vi "DPT Call.vi"() -> ()   [LabVIEW 2014]
panel:
  in  "Source Library Path":path=path "\\\\192.168.1.12\\share/AP1_Library/Executables/Dryer Performance Test"
  out "Array 2":bool[](array[boolean])=[TRUE, TRUE, TRUE, TRUE]
  out "Error Array":errorcluster[](array[cluster])
  out "Response":string[](array[string])
  out "Cmd":i32
  in  "error in (no error)":errorcluster
  out "Cmds Array":string[](array[string])
  in  "configuration file path":path=path "C:/work/DryerPerformanceTest.ini"
  in  "data backup command line":string="robocopy \"c:\\Data\" \"XXX\"  /XN"
  in  "update command line":string="robocopy \"XXX\"  \"c:\\Program Files\\GE\\Dryer Performance Test\" /XN"
  in  "backup command line":string="robocopy \"c:\\Program Files\\GE\\Dryer Performance Test\"  \"c:\\Program Files\\GE\\backup\" /XN"
  out "error out":errorcluster
  in  "command line":string="\"c:\\Program Files\\GE\\Dryer Performance Test\\Dryer Performance Test.exe\""
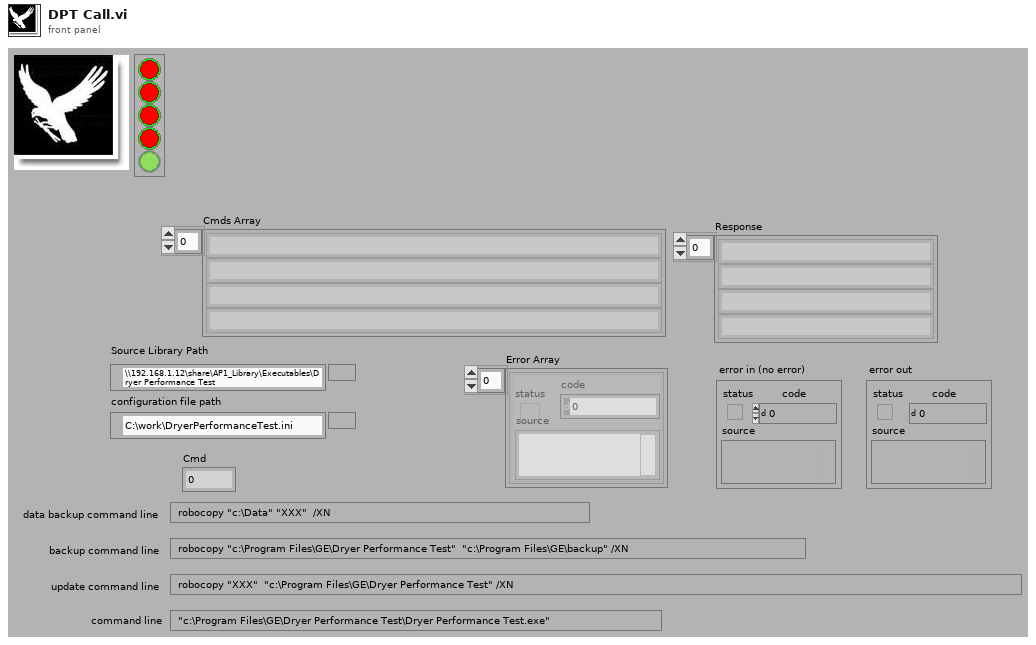
[diagram p1: front panel]
types:
  T1 = typedef "DPT Global Type.ctl" = cluster{"Test Setup":cluster{"RH Resistor":dbl, "Temp Cal":dbl, "Temp Coeff":dbl, "Power On Threshold":dbl, "MA Filter Size":i32, "Weight Offset":dbl, "Temp Resistor":dbl, "Gas Enabled":bool, "Gas P. Resistor":dbl, "Scale Com":dbl, "W. Samps":i32, "Temp4mA Val":dbl, "Temp20mA Val":dbl, "RH4mA Val":dbl, "RH20mA Val":dbl, "GPres4mA Val":dbl, "Gpres20mA Val":dbl, "Smoothing":bool, "CDAQ":bool, "34970":bool, "34980":bool, "RH-IP":string, "RH-IP2":string, "RH-IP3":string, "CompVolume":dbl, "T45_Coeff.":dbl}, "Agilent Setup":cluster{"Scale Channel":string, "TC Channels":string, "VDC Discrete Channels":string, "RH Chan":string, "Temp Chan":string, "Tscale Channel":string, "RDB Channel":string, "Gas Temperature":string, "Gas Pressure":string, "Barometric Pressure":string, "Gas Feedback Chan":string}, "Directories":cluster{"Work File Directory":path, "Save File Directory":path, "Library Directory":path, "Data Backup Directory":path, "Data Backup Dir Fail":path, "Lab Directory":path}, "Test Information":cluster{"Model:":string, "Temperature:":string, "Engineer:":string, "Technician:":string, "Comments:":string, "Lab ID:":string, "TR Number:":string, "Test Number:":string, "Test Station:":string, "Empty Dryer Cold Weight:":dbl, "Serial Number:":string, "Build:":string, "Dryer Type":string, "Humidity":string, "Test Title per TR:":string}, "cDAQ Array Locations":cluster{"Scale Channel":string, "TC Channels":string, "VDC Discrete Channel":string, "RH Chan":string, "Temp Chan":string, "Tscale Channel":string, "RDB Channel":string, "Gas Temperature":string, "Gas Pressure":string, "Barometric Pressure":string, "Gas Feedback Chan":string}}
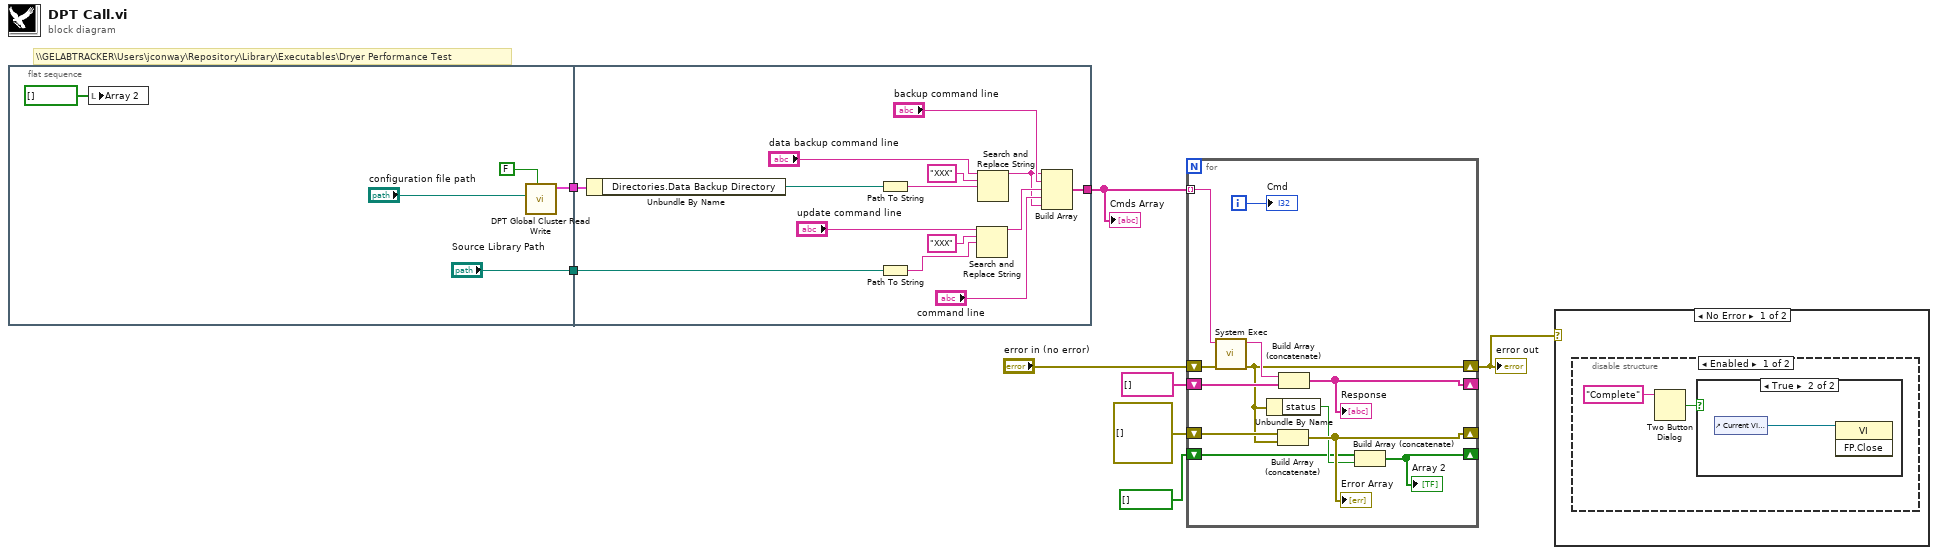
[diagram p0: block diagram]
diagram:
  # "\\\\GELABTRACKER\\Users\\jconway\\Repository\\Library\\Executables\\Dryer Performance Test"
  n1 = flat-sequence {
    tunnel: [w13] -> w7
    tunnel: ["Source Library Path"] -> w1
    tunnel: [w26] -> w8
    tunnel: w7 -> [w23]
    tunnel: w1 -> [w14]
    frame #0 {
      n2 = local write "Array 2"(bool[] [] ("Array 2")) -> ()
      n3 = call "DPT Global Cluster Read Write.vi"("Write?"=FALSE, "configuration file path"="configuration file path") -> ("Test Config Out"=w13:T1)  [unwired: 8 in, 1 out]
    }
    frame #1 {
      n4 = Unbundle By Name(w23) -> ("Directories.Data Backup Directory"=w25:path)
      n5 = Path To String(path=w25) -> (string=w24:string)
      n6 = Path To String(path=w14) -> (string=w20:string)
      n7 = Search and Replace String(input string="update command line", search string="XXX", replace string=w20) -> (result string=w16:string)  [unwired: 5 in, 3 out]
      n8 = Search and Replace String(input string="data backup command line", search string="XXX", replace string=w24) -> (result string=w15:string)  [unwired: 5 in, 3 out]
      n9 = Build Array(w15, "backup command line", w16, "command line", w15) -> (w26:string[])
    }
  }
  n10 = for {
    tunnel: w8 -> [w39] mode=indexing
    shift-right: [w32] -> w5
    shift-left: "error in (no error)" -> [w38]
    shift-right: [w34] -> _
    shift-left: string[] [] -> [w35]
    shift-right: [w31] -> _
    shift-left: errorcluster[] [] -> [w33]
    shift-right: [w28] -> _
    shift-left: bool[] [] -> [w29]
    i -> [w37]
    n11 = call <vilib>:"System Exec.vi"("error in (no error)"=w38, "command line"=w39) -> ("error out"=w32:errorcluster, "standard output"=w36:string)  [unwired: 6 in, 2 out]
    n12 = Unbundle By Name(w32) -> ("status"=w30:bool)
    n13 = Build Array (concatenate)(w33, w32) -> (w31:errorcluster[])
    "Error Array" <- w31
    n14 = Build Array (concatenate)(w36, w35) -> (w34:string[])
    "Response" <- w34
    n15 = Build Array (concatenate)(w29, w30) -> (w28:bool[])
    "Array 2" <- w28
    "Cmd" <- w37
  }
  "error out" <- w5
  n16 = case shown="No Error" w5 {
    frame No Error {
      n17 = disable-structure shown="Enabled" {
        frame Enabled {
          n18 = Two Button Dialog(message="Complete") -> (T button?=w41:bool)  [unwired: 2 in]
          n19 = case shown="True" w41 {
            frame False {
            }
            frame True {
              n20 = control-ref of="Current VI Reference"() -> (w42:refnum<vi>)
              n21 = invoke class="VI" method="FP.Close"(reference=w42) -> ()  [unwired: 2 in, 3 out]
            }
          }
        }
        frame Disabled {
        }
      }
    }
    frame Error {
    }
  }
  "Cmds Array" <- w8
